vi "IN Range check.vi"(5 "UL":dbl, 7 "Data Point":dbl, 9 "LL":dbl) -> (8 "In range ?":bool)   [LabVIEW 2020]
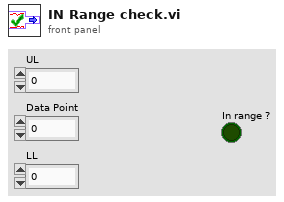
[diagram p1: front panel]
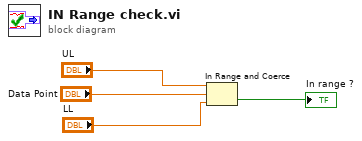
[diagram p0: block diagram]
diagram:
  n1 = In Range and Coerce(upper limit="UL", x="Data Point", lower limit="LL") -> (In Range?=→"In range ?":bool)  [unwired: 1 out]
